vi "test-cubic-spline-04B.vi"() -> (3 "Test Passed":bool)   [LabVIEW 2019]
uses:
  <vilib>/Rock Robotics/WPI/ThirdParty/JAS_Junk/TrajLib/POSEwCURVATURE.ctl
  <vilib>/Rock Robotics/WPI/ThirdParty/JAS_Junk/TrajLib/POSE2D.ctl
  <vilib>/Rock Robotics/WPI/ThirdParty/JAS_Junk/TrajLib/TRANSLATION2D.ctl
  <vilib>/Rock Robotics/WPI/ThirdParty/JAS_Junk/TrajLib/ROTATION2D.ctl
  <vilib>/Rock Robotics/WPI/ThirdParty/JAS_Junk/TrajLib/Rotation_CreateAngle.vi
  <vilib>/Rock Robotics/WPI/ThirdParty/JAS_Junk/TrajLib/Util_CalcDist.vi
  <vilib>/Rock Robotics/WPI/ThirdParty/JAS_Junk/TrajLib/Trajectory_Library.lvlib
panel:
  out "XY Graph":cluster{dbl[], dbl[]}(graph)
  out "All Interior \nwayPoints\nFound (True)":bool
  out "end rot = 0":dbl
  out "end y = 0":dbl
  out "end x = 0":dbl
  out "start rot = 0":dbl
  out "start y = 0":dbl
  out "start x = 0":dbl
  out "max dtheta < 0.0872":dbl
  out "max dy < 0.00127":dbl
  out "max dx  < 0.127":dbl
  out "Overall Error":errorcluster
  out "Elements":i32
  out "Create Spline Error":errorcluster
  out "SplinePoses\nWCurve":T1[](array[typedef]) {"POSE"."ROTATION"."SIN" format="%13.4f"; "POSE"."ROTATION"."COS" format="%13.4f"; "POSE"."ROTATION"."VALUE" format="%13.4f"; "POSE"."TRANSLATION"."Y" format="%14.3f"; "POSE"."TRANSLATION"."X" format="%14.3f"}
  out "Elapsed Time":dbl
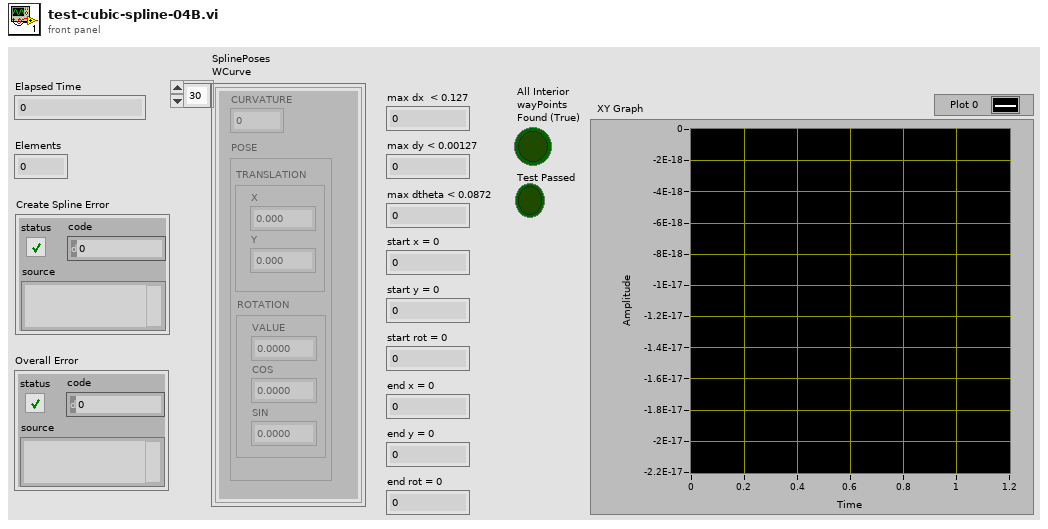
[diagram p1: front panel]
types:
  T1 = typedef "Trajectory_Library.lvlib/POSEwCURVATURE.ctl" = cluster{"CURVATURE":dbl, "POSE":T2}
  T2 = typedef "Trajectory_Library.lvlib/POSE2D.ctl" = cluster{"TRANSLATION":T3, "ROTATION":T4}
  T3 = typedef "Trajectory_Library.lvlib/TRANSLATION2D.ctl" = cluster{"X":dbl, "Y":dbl}
  T4 = typedef "Trajectory_Library.lvlib/ROTATION2D.ctl" = cluster{"VALUE":dbl, "COS":dbl, "SIN":dbl}
  T5 = typedef "Trajectory_Library.lvlib/SPLINE_CTRL_VECTOR.ctl" = cluster{"Xs":dbl[], "Ys":dbl[]}
  T6 = typedef "Trajectory_Library.lvlib/SPLINE.ctl" = cluster{"Degree":i32, "Coefficients":T7}
  T7 = typedef "NI_Matrix.lvlib/RealMatrix.ctl" = dbl[][]
  T8 = typedef "Trajectory_Library.lvlib/TWIST2D.ctl" = cluster{"dX":dbl, "dY":dbl, "dTHETA":dbl}
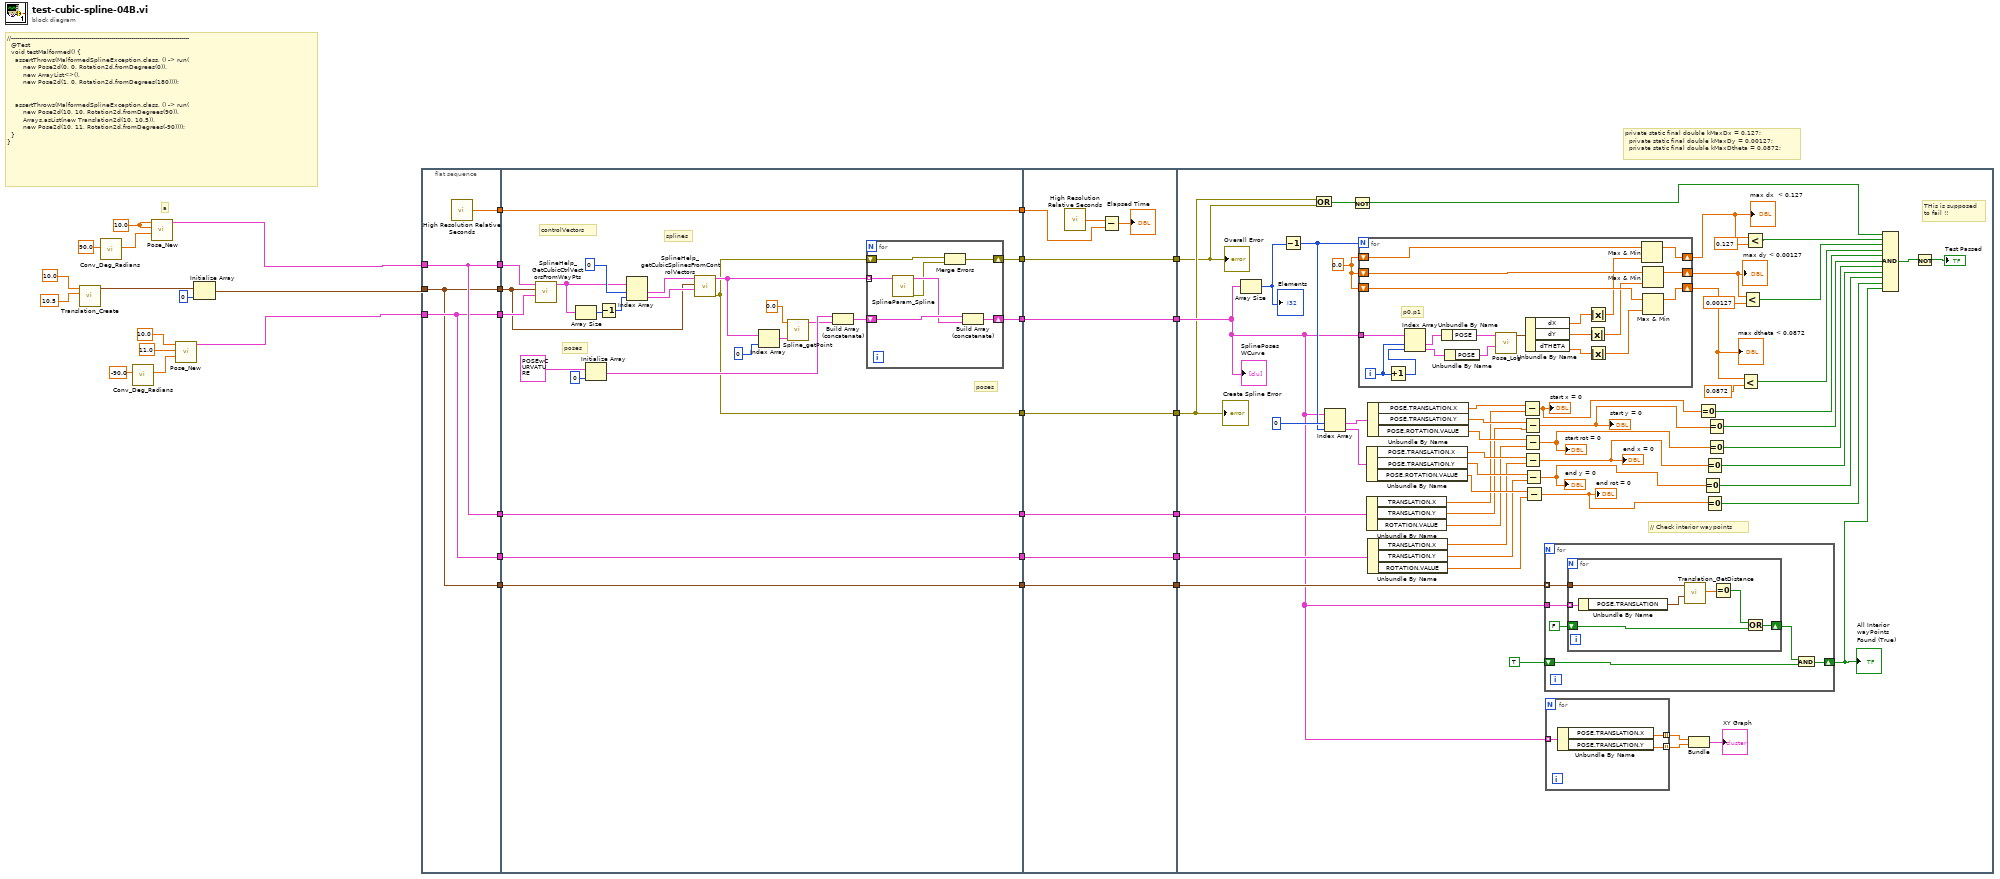
[diagram p0: block diagram]
diagram:
  w12 = 10.0 ("X")
  # "a"
  # "//-----------------------------------------------------------------------------------------\n  @Test\n  void testMalformed() {\n    assertThrows(MalformedSplineException.class, () -> run(\n        new Pose2d(0, 0, Rotation2d.fromDegrees(0)),\n        new ArrayList<>(), \n        new Pose2d(1, 0, Rotation2d.fromDegrees(180))));\n\n\n    assertThrows(MalformedSplineException.class, () -> run(\n        new Pose2d(10, 10, Rotation2d.fromDegrees(90)),\n        Arrays.asList(new Translation2d(10, 10.5)),\n        new Pose2d(10, 11, Rotation2d.fromDegrees(-90))));\n  }\n}"
  # "private static final double kMaxDx = 0.127;\n  private static final double kMaxDy = 0.00127;\n  private static final double kMaxDtheta = 0.0872;"
  n1 = call <vilib>:"Translation_Create.vi"("Y"=10.5, "X"=10.0) -> ("TRANSLATION"=w1:T3)  [unwired: 9 in]
  n2 = call <vilib>:"Conv_Deg_Radians.vi"("Degress"=90.0) -> ("Radians"=w11:dbl)  [unwired: 10 in]
  n3 = call <vilib>:"Conv_Deg_Radians.vi"("Degress"=-90.0) -> ("Radians"=w8:dbl)  [unwired: 10 in]
  n4 = call <vilib>:"Pose_New.vi"("Heading"=w11, "Y"=w12, "X"=w12) -> ("out POSe"=w6:T2)  [unwired: 8 in]
  n5 = call <vilib>:"Pose_New.vi"("Heading"=w8, "Y"=11.0, "X"=10.0) -> ("out POSe"=w4:T2)  [unwired: 8 in]
  n6 = Initialize Array(w1, 0 ("dimension size")) -> (w5:T3[])
  n7 = flat-sequence {
    tunnel: w6 -> [w37]
    tunnel: [w37] -> w34
    tunnel: w5 -> [w35]
    tunnel: [w35] -> w33
    tunnel: w4 -> [w36]
    tunnel: [w36] -> w32
    tunnel: [w38] -> w31
    tunnel: [w37] -> w23
    tunnel: [w36] -> w20
    tunnel: [w35] -> w15
    tunnel: w34 -> [w63]
    tunnel: w33 -> [w55]
    tunnel: w32 -> [w62]
    tunnel: [w54] -> w30
    tunnel: w31 -> [w54]
    tunnel: [w44] -> w29
    tunnel: [w43] -> w27
    tunnel: [w42] -> w25
    tunnel: w23 -> [w41]
    tunnel: [w41] -> w22
    tunnel: w20 -> [w40]
    tunnel: [w40] -> w19
    tunnel: [w39] -> w16
    tunnel: w15 -> [w39]
    tunnel: w30 -> [w79]
    tunnel: w29 -> [w78]
    tunnel: [w78] -> w28
    tunnel: w27 -> [w77]
    tunnel: [w77] -> w26
    tunnel: w25 -> [w76]
    tunnel: [w76] -> w24
    tunnel: w22 -> [w73]
    tunnel: [w73] -> w21
    tunnel: w19 -> [w72]
    tunnel: [w72] -> w18
    tunnel: [w71] -> w17
    tunnel: w16 -> [w71]
    tunnel: w28 -> [w108]
    tunnel: w26 -> [w84]
    tunnel: w24 -> [w83]
    tunnel: w21 -> [w131]
    tunnel: w18 -> [w130]
    tunnel: w17 -> [w113]
    frame #0 {
      n8 = call <vilib>:"High Resolution Relative Seconds.vi"() -> ("relative seconds"=w38:dbl)
    }
    frame #1 {
      # "poses"
      # "poses"
      # "splines"
      # "controlVectors"
      n9 = call <vilib>:"SplineHelp_GetCubicCtrlVectorsFromWayPts.vi"("Enging POSE"=w62, "Interior WAYPOINTS"=w55, "Starting POSE"=w63) -> ("SplineControlVectors"=w59:T5[])  [unwired: 8 in]
      n10 = Array Size(array=w59) -> (size(s)=w60:i32)
      n11 = Initialize Array(T1 {"CURVATURE"=0.0, "POSE"={"TRANSLATION"={"X"=0.0, "Y"=0.0}, "ROTATION"={"VALUE"=0.0, "COS"=1.0, "SIN"=0.0}}} ("POSEwCURVATURE"), 0 ("dimension size")) -> (w48:T1[])
      n12 = Decrement(x=w60) -> (x-1=w58:i32)
      n13 = Index Array(array=w59, index #1=0 ("index"), index #2=w58) -> (element #1=w57:T5, element #2=w56:T5)
      n14 = call <vilib>:"SplineHelp_getCubicSplinesFromControlVectors.vi"("endCtrlVector"=w56, "InternalWaypoints"=w55, "startCtrlVector"=w57) -> ("error out"=w43:errorcluster, "splines"=w45:T6[])  [unwired: 3 in, 4 out]
      n15 = Index Array(array=w45, index=0) -> (element=w50:T6)
      n16 = call <vilib>:"Spline_getPoint.vi"("inputSPLINE"=w50, "Time"=0.0) -> ("POSEwCURVATURE"=w47:T1)  [unwired: 9 in]
      n17 = Build Array (concatenate)(w48, w47) -> (w46:T1[])
      n18 = for {
        shift-right: [w67] -> w44
        shift-left: w46 -> [w69]
        tunnel: w45 -> [w70] mode=indexing
        shift-right: [w65] -> w42
        shift-left: w43 -> [w66]
        n19 = call <vilib>:"SplineParam_Spline.vi"("inputSPLINE"=w70) -> ("error out"=w64:errorcluster, "outputPOSEwCURVATURE"=w68:T1[])  [unwired: 9 in]
        n20 = Merge Errors(w66, w64) -> (w65:errorcluster)
        n21 = Build Array (concatenate)(w69, w68) -> (w67:T1[])
      }
    }
    frame #2 {
      n22 = call <vilib>:"High Resolution Relative Seconds.vi"() -> ("relative seconds"=w74:dbl)
      n23 = Subtract(x=w74, y=w79) -> (x-y=→"Elapsed Time":dbl)
    }
    frame #3 {
      w132 = 0.0
      # "THis is supposed\nto fail !!"
      # "// Check interior waypoints"
      n24 = Array Size(array=w108) -> (size(s)=w133:i32)
      "Elements" <- w133
      n25 = Decrement(x=w133) -> (x-1=w128:i32)
      n26 = Or(x=w84, y=w83) -> (x .or. y?=w85:bool)
      n27 = Index Array(array=w108, index #1=0 ("index"), index #2=w128) -> (element #1=w127:T1, element #2=w126:T1)
      n28 = Not(x=w85) -> (.not. x?=w82:bool)
      n29 = for {
        N: w128 -> [_]
        tunnel: w108 -> [w167]
        shift-right: [w158] -> w105
        shift-left: w132 -> [w155]
        shift-right: [w156] -> w107
        shift-left: w132 -> [w153]
        shift-right: [w157] -> w106
        shift-left: w132 -> [w154]
        i -> [w169]
        # "p0,p1"
        n30 = Increment(x=w169) -> (x+1=w168:i32)
        n31 = Index Array(array=w167, index #1=w169, index #2=w168) -> (element #1=w166:T1, element #2=w165:T1)
        n32 = Unbundle By Name(w166) -> ("POSE"=w164:T2)
        n33 = Unbundle By Name(w165) -> ("POSE"=w163:T2)
        n34 = call <vilib>:"Pose_Log.vi"("end POSE"=w163, "in POSE"=w164) -> ("out TWIST"=w162:T8)  [unwired: 9 in]
        n35 = Unbundle By Name(w162) -> ("dX"=w159:dbl, "dY"=w160:dbl, "dTHETA"=w161:dbl)
        n36 = Absolute Value(x=w160) -> (abs(x)=w151:dbl)
        n37 = Absolute Value(x=w159) -> (abs(x)=w152:dbl)
        n38 = Absolute Value(x=w161) -> (abs(x)=w150:dbl)
        n39 = Max & Min(x=w155, y=w152) -> (max(x,y)=w158:dbl)  [unwired: 1 out]
        n40 = Max & Min(x=w154, y=w151) -> (max(x,y)=w157:dbl)  [unwired: 1 out]
        n41 = Max & Min(x=w153, y=w150) -> (max(x,y)=w156:dbl)  [unwired: 1 out]
      }
      "max dx  < 0.127" <- w105
      "max dy < 0.00127" <- w106
      "max dtheta < 0.0872" <- w107
      n42 = Unbundle By Name(w126) -> ("POSE.TRANSLATION.X"=w122:dbl, "POSE.TRANSLATION.Y"=w121:dbl, "POSE.ROTATION.VALUE"=w120:dbl)
      n43 = Unbundle By Name(w131) -> ("TRANSLATION.X"=w119:dbl, "TRANSLATION.Y"=w118:dbl, "ROTATION.VALUE"=w117:dbl)
      n44 = Unbundle By Name(w127) -> ("POSE.TRANSLATION.X"=w125:dbl, "POSE.TRANSLATION.Y"=w124:dbl, "POSE.ROTATION.VALUE"=w123:dbl)
      n45 = Unbundle By Name(w130) -> ("TRANSLATION.X"=w116:dbl, "TRANSLATION.Y"=w115:dbl, "ROTATION.VALUE"=w114:dbl)
      n46 = Subtract(x=w125, y=w119) -> (x-y=w98:dbl)
      "start x = 0" <- w98
      n47 = Subtract(x=w124, y=w118) -> (x-y=w97:dbl)
      "start y = 0" <- w97
      n48 = Subtract(x=w123, y=w117) -> (x-y=w96:dbl)
      "start rot = 0" <- w96
      n49 = Subtract(x=w122, y=w116) -> (x-y=w95:dbl)
      "end x = 0" <- w95
      n50 = Subtract(x=w121, y=w115) -> (x-y=w94:dbl)
      "end y = 0" <- w94
      n51 = Subtract(x=w120, y=w114) -> (x-y=w93:dbl)
      "end rot = 0" <- w93
      n52 = for {
        tunnel: w113 -> [w137] mode=indexing
        tunnel: w108 -> [w142]
        shift-right: [w141] -> w86
        shift-left: TRUE -> [w140]
        n53 = for {
          tunnel: w142 -> [w146] mode=indexing
          shift-right: [w149] -> w138
          shift-left: FALSE -> [w148]
          tunnel: w137 -> [w147]
          n54 = Unbundle By Name(w146) -> ("POSE.TRANSLATION"=w145:T3)
          n55 = call <vilib>:"Translation_GetDistance.vi"("other Translation"=w145, "In Translation"=w147) -> ("Distance"=w144:dbl)  [unwired: 9 in]
          n56 = Equal To 0?(x=w144) -> (x = 0?=w143:bool)
          n57 = Or(x=w143, y=w148) -> (x .or. y?=w149:bool)
        }
        n58 = And(x=w138, y=w140) -> (x .and. y?=w141:bool)
      }
      "All Interior \nwayPoints\nFound (True)" <- w86
      n59 = for {
        tunnel: [w136] -> w111 mode=indexing
        tunnel: [w135] -> w110 mode=indexing
        tunnel: w108 -> [w134] mode=indexing
        n60 = Unbundle By Name(w134) -> ("POSE.TRANSLATION.X"=w136:dbl, "POSE.TRANSLATION.Y"=w135:dbl)
      }
      n61 = Bundle(w111, w110) -> (→"XY Graph":cluster{dbl[], dbl[]})  [unwired: 1 in]
      n62 = Equal To 0?(x=w98) -> (x = 0?=w92:bool)
      n63 = Equal To 0?(x=w94) -> (x = 0?=w88:bool)
      n64 = Equal To 0?(x=w95) -> (x = 0?=w89:bool)
      n65 = Equal To 0?(x=w93) -> (x = 0?=w87:bool)
      n66 = Equal To 0?(x=w97) -> (x = 0?=w91:bool)
      n67 = Equal To 0?(x=w96) -> (x = 0?=w90:bool)
      n68 = Less?(x=w107, y=0.0872) -> (x < y?=w99:bool)
      n69 = Less?(x=w106, y=0.00127) -> (x < y?=w100:bool)
      n70 = Less?(x=w105, y=0.127) -> (x < y?=w101:bool)
      n71 = Compound Arithmetic op=AND(w82, w101, w100, w99, w92, w91, w90, w89, w88, w87, w86) -> (w80:bool)
      n72 = Not(x=w80) -> (.not. x?=→"Test Passed":bool)
      "SplinePoses\nWCurve" <- w108
      "Create Spline Error" <- w84
      "Overall Error" <- w83
    }
  }
